vi "Write Polling Period, ms.vi"(8 "error in (no error)":errorcluster, 10 "Polling Period, ms":i64=-1, 11 "Base Hardware in":refnum<class "Base Hardware.lvclass">) -> (0 "error out":errorcluster, 3 "Base Hardware out":refnum<class "Base Hardware.lvclass">)   [LabVIEW 2023, in "Abstract Hardware.lvlib" / "Base Hardware.lvclass"]
uses:
  Base Hardware.lvclass
  Base Hardware.lvclass/Base Hardware.ctl
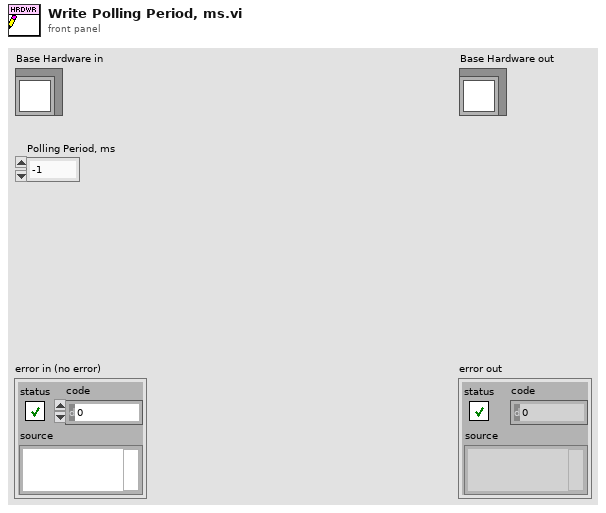
[diagram p1: front panel]
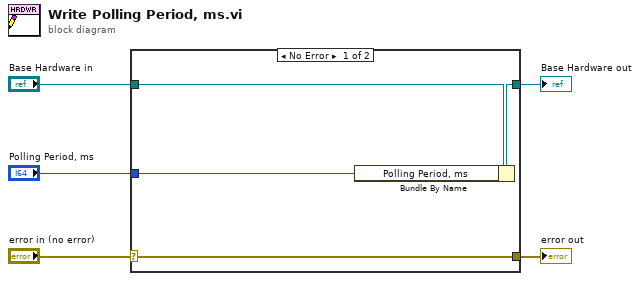
[diagram p0: block diagram]
diagram:
  n1 = case shown="No Error" "error in (no error)" {
    selector: "error in (no error)" -> [w9 w10]
    tunnel: [w9 w10] -> w4
    tunnel: [w7 w11] -> w2
    tunnel: "Base Hardware in" -> [w8 w11]
    tunnel: "Polling Period, ms" -> [w6 _]
    frame No Error {
      n2 = Bundle By Name(cluster=w8, "Polling Period, ms"=w6) -> (w7:refnum<class "Base Hardware.lvclass">)
    }
    frame Error {
    }
  }
  "error out" <- w4
  "Base Hardware out" <- w2
